vi "ChannelType_2D-Array-U64_Color.vi"(9 "error in":errorcluster, 11 "Array in":u64[][](array[numeric])) -> (1 "error out":errorcluster, 2 "ChannelType":u16, 3 "Array out":u64[][](array[numeric]))   [LabVIEW 2020, in "OpenLvVision_OpenCv.lvlib"]
uses:
  OpenLvVision_OpenCv.lvlib
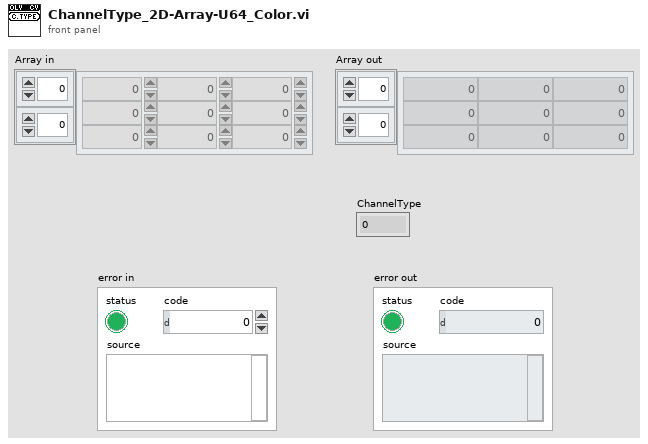
[diagram p1: front panel]
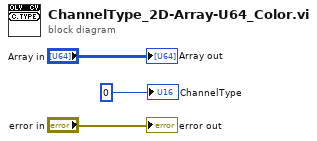
[diagram p0: block diagram]
diagram:
  "error out" <- "error in"
  "Array out" <- "Array in"
  "ChannelType" <- u16 0
